vi "Part 2.vi"(11 "Input":string) -> (3 "Output":i64)   [LabVIEW 2021]
uses:
  <userlib>/_OpenG.lib/string/string.llb/Convert EOLs (String)__ogtk.vi
panel:
  in  "Numeric":i32=1
  out "Array":i64[](array[numeric])
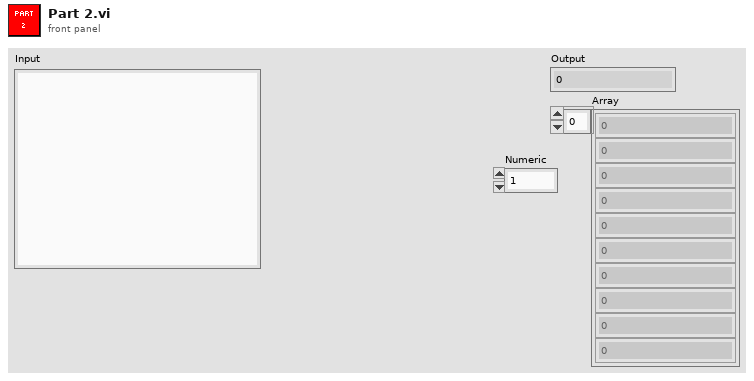
[diagram p1: front panel]
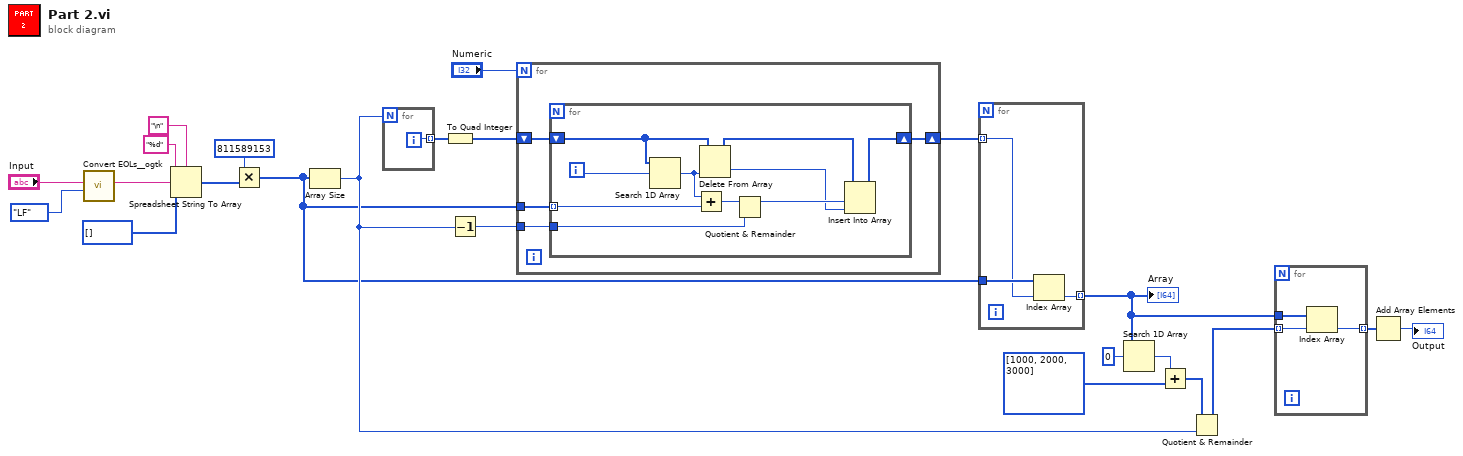
[diagram p0: block diagram]
diagram:
  n1 = call-poly <userlib>:"Convert EOLs__ogtk.vi"("Convert to:"=enum16{"CR", "LF", "CRLF"}."LF", "String in"="Input") -> ("String out"=w19:string)  [unwired: 9 in]
  n2 = Spreadsheet String To Array(delimiter (Tab)="\n", format string="%d", spreadsheet string=w19, array type (2D Dbl)=i64[] []) -> (array=w15:i64[])
  n3 = Multiply(x=i64 811589153, y=w15) -> (x*y=w3:i64[])
  n4 = Array Size(array=w3) -> (size(s)=w11:i32)
  n5 = for {
    N: w11 -> [_]
    tunnel: [w24] -> w10 mode=indexing
    i -> [w24]
  }
  n6 = To Quad Integer(1:w10) -> (0:w9:i64[])
  n7 = Decrement(x=w11) -> (x-1=w17:i32)
  n8 = for {
    N: "Numeric" -> [_]
    tunnel: w17 -> [w28]
    tunnel: w3 -> [w25]
    shift-right: [w26] -> w8
    shift-left: w9 -> [w27]
    n9 = for {
      tunnel: w25 -> [w38] mode=indexing
      shift-right: [w30] -> w26
      shift-left: w27 -> [w32]
      tunnel: w28 -> [w29]
      i -> [w34]
      n10 = Search 1D Array(1D array=w32, element=w34) -> (index of element=w37:i32)  [unwired: 1 in]
      n11 = Add(x=w37, y=w38) -> (x+y=w36:i64)
      n12 = Delete From Array(array=w32, index=w37) -> (deleted portion=w33:i64, array with subset deleted=w31:i64[])  [unwired: 1 in]
      n13 = Quotient & Remainder(x=w36, y=w29) -> (x-y*floor(x/y)=w35:i64)  [unwired: 1 out]
      n14 = Insert Into Array(array=w31, index=w35, new element=w33) -> (w30:i64[])
    }
  }
  n15 = for {
    tunnel: w8 -> [w40] mode=indexing
    tunnel: w3 -> [w41]
    tunnel: [w39] -> w4 mode=indexing
    n16 = Index Array(array=w41, index=w40) -> (element=w39:i64)
  }
  "Array" <- w4
  n17 = Search 1D Array(1D array=w4, element=i64 0) -> (index of element=w7:i32)  [unwired: 1 in]
  n18 = Add(x=w7, y=i64[] [1000, 2000, 3000]) -> (x+y=w6:i64[])
  n19 = Quotient & Remainder(x=w6, y=w11) -> (x-y*floor(x/y)=w5:i64[])  [unwired: 1 out]
  n20 = for {
    tunnel: w4 -> [w44]
    tunnel: w5 -> [w43] mode=indexing
    tunnel: [w42] -> w13 mode=indexing
    n21 = Index Array(array=w44, index=w43) -> (element=w42:i64)
  }
  n22 = Add Array Elements(numeric array=w13) -> (sum=→"Output":i64)
